vi "single_move.vi"(0 "COM In":refnum<visa-resource-name>, 1 "error In":errorcluster caption="error out", 2 "速度(r/min)":u16=60, 3 "反向":bool=TRUE, 4 "移动距离(mm)":dbl=2.0 caption="元素", 7 "Y轴":bool=TRUE, 8 "细分":u16=40000) -> (5 "VISA resource name out 2":refnum<visa-resource-name>, 6 "error out 2":errorcluster caption="error out")   [LabVIEW 2018]
uses:
  location_x.vi
  location_y.vi
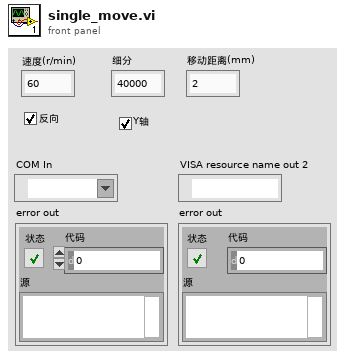
[diagram p1: front panel]
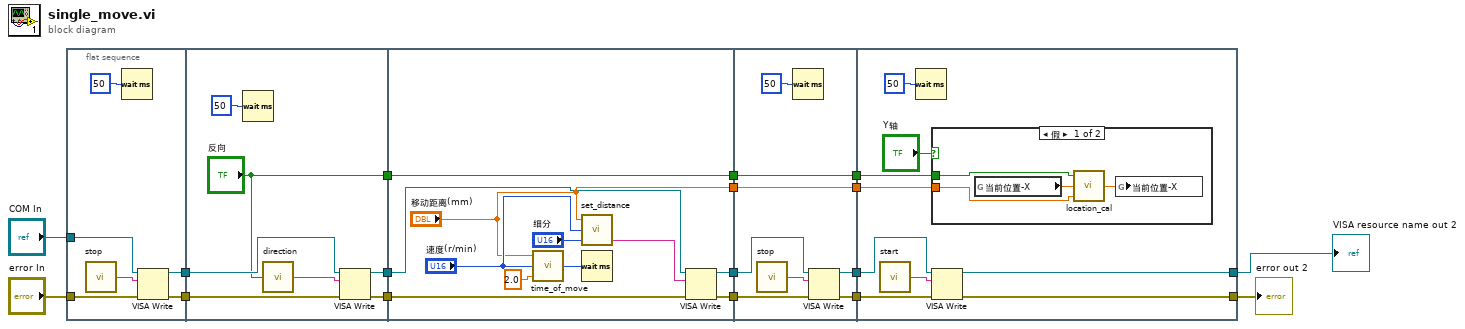
[diagram p0: block diagram]
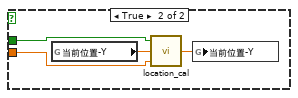
[diagram p2: hidden frame]
diagram:
  n1 = flat-sequence {
    tunnel: "error In" -> [w22]
    tunnel: "COM In" -> [w21]
    tunnel: [w20] -> w7
    tunnel: [w19] -> w6
    tunnel: [w29] -> w17
    tunnel: [w30] -> w16
    tunnel: w7 -> [w26]
    tunnel: w6 -> [w25]
    tunnel: ["反向"] -> w3
    tunnel: [w38] -> w15
    tunnel: [w40] -> w14
    tunnel: w17 -> [w39]
    tunnel: w16 -> [w41]
    tunnel: [w32] -> w4
    tunnel: w3 -> [w32]
    tunnel: ["移动距离(mm)"] -> w1
    tunnel: [w46] -> w13
    tunnel: [w48] -> w12
    tunnel: w15 -> [w47]
    tunnel: w14 -> [w49]
    tunnel: [w43] -> w5
    tunnel: w4 -> [w43]
    tunnel: [w42] -> w2
    tunnel: w1 -> [w42]
    tunnel: [w56] -> w8
    tunnel: [w55] -> w9
    tunnel: w13 -> [w58]
    tunnel: w12 -> [w57]
    tunnel: w5 -> [w51]
    tunnel: w2 -> [w50]
    frame #0 {
      n2 = call "stop.vi"() -> ("指令"=w23:string)
      n3 = Wait (ms)(milliseconds to wait=u32 50 ("等待时间（毫秒）")) -> ()  [unwired: 1 out]
      n4 = VISA Write(VISA resource name=w21, write buffer=w23, error in (no error)=w22) -> (VISA resource name out=w20:refnum<visa-resource-name>, error out=w19:errorcluster)  [unwired: 1 out]
    }
    frame #1 {
      n5 = Wait (ms)(milliseconds to wait=u32 50 ("等待时间（毫秒）")) -> ()  [unwired: 1 out]
      n6 = call "direction.vi"("反向"="反向") -> ("指令"=w28:string)
      n7 = VISA Write(VISA resource name=w26, write buffer=w28, error in (no error)=w25) -> (VISA resource name out=w30:refnum<visa-resource-name>, error out=w29:errorcluster)  [unwired: 1 out]
    }
    frame #2 {
      n8 = call "time_of_move.vi"("导程"=2.0, "转速"="速度(r/min)", "移动距离"="移动距离(mm)") -> ("所需时间"=w33:i32)
      n9 = call "set_distance.vi"("细分"="细分", "速度(r/min)"="速度(r/min)", "移动距离(mm)"="移动距离(mm)") -> ("指令"=w37:string)  [unwired: 2 out]
      n10 = Wait (ms)(milliseconds to wait=w33) -> ()  [unwired: 1 out]
      n11 = VISA Write(VISA resource name=w41, write buffer=w37, error in (no error)=w39) -> (VISA resource name out=w40:refnum<visa-resource-name>, error out=w38:errorcluster)  [unwired: 1 out]
    }
    frame #3 {
      n12 = call "stop.vi"() -> ("指令"=w45:string)
      n13 = Wait (ms)(milliseconds to wait=u32 50 ("等待时间（毫秒）")) -> ()  [unwired: 1 out]
      n14 = VISA Write(VISA resource name=w49, write buffer=w45, error in (no error)=w47) -> (VISA resource name out=w48:refnum<visa-resource-name>, error out=w46:errorcluster)  [unwired: 1 out]
    }
    frame #4 {
      n15 = call "start.vi"() -> ("指令"=w54:string)
      n16 = Wait (ms)(milliseconds to wait=u32 50 ("等待时间（毫秒）")) -> ()  [unwired: 1 out]
      n17 = case shown="假" "Y轴" {
        tunnel: w51 -> [w61 w65]
        tunnel: w50 -> [w59 w63]
        frame False {
          n18 = global read "location_x.vi" "当前位置-X"() -> (w62:dbl)
          n19 = call "location_cal.vi"("移动距离"=w59, "当前位置"=w62, "反向"=w61) -> ("结束位置"=w60:dbl)
          n20 = global write "location_x.vi" "当前位置-X"(w60) -> ()
        }
        frame True {
          n21 = global read "location_y.vi" "当前位置-Y"() -> (w66:dbl)
          n22 = call "location_cal.vi"("移动距离"=w63, "当前位置"=w66, "反向"=w65) -> ("结束位置"=w64:dbl)
          n23 = global write "location_y.vi" "当前位置-Y"(w64) -> ()
        }
      }
      n24 = VISA Write(VISA resource name=w57, write buffer=w54, error in (no error)=w58) -> (VISA resource name out=w55:refnum<visa-resource-name>, error out=w56:errorcluster)  [unwired: 1 out]
    }
  }
  "VISA resource name out 2" <- w9
  "error out 2" <- w8
